vi "GetSegmentBands.vi"(9 "stop frequency":dbl format="%#_6p", 10 "start frequency":dbl format="%#_6p", 11 "sweeps in":T1[](array[typedef]) {"bandwidth" format="%#_6p"; "stop" format="%#_6p"; "start" format="%#_6p"}) -> (3 "sweeps out":T1[](array[typedef]) {"bandwidth" format="%#_6p"; "stop" format="%#_6p"; "start" format="%#_6p"})   [LabVIEW 2017, in "EmsaAnalysis.lvlib"]
uses:
  <vilib>/addons/InsightCM/Devices/Shared/Emsa/EmsaAnalysis/EmsaAnalysis.lvlib
  <vilib>/addons/InsightCM/Devices/Shared/Emsa/EmsaAnalysis/controls/sweepInfo.ctl
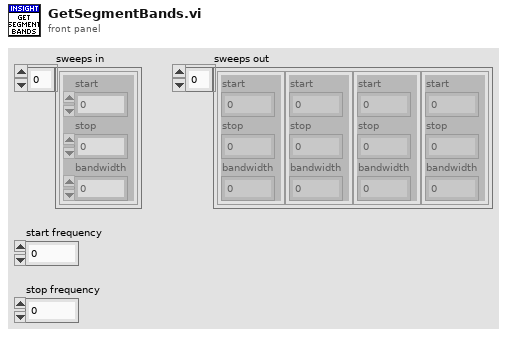
[diagram p1: front panel]
types:
  T1 = typedef "EmsaAnalysis.lvlib/sweepInfo.ctl" = cluster{"start":dbl, "stop":dbl, "bandwidth":dbl}
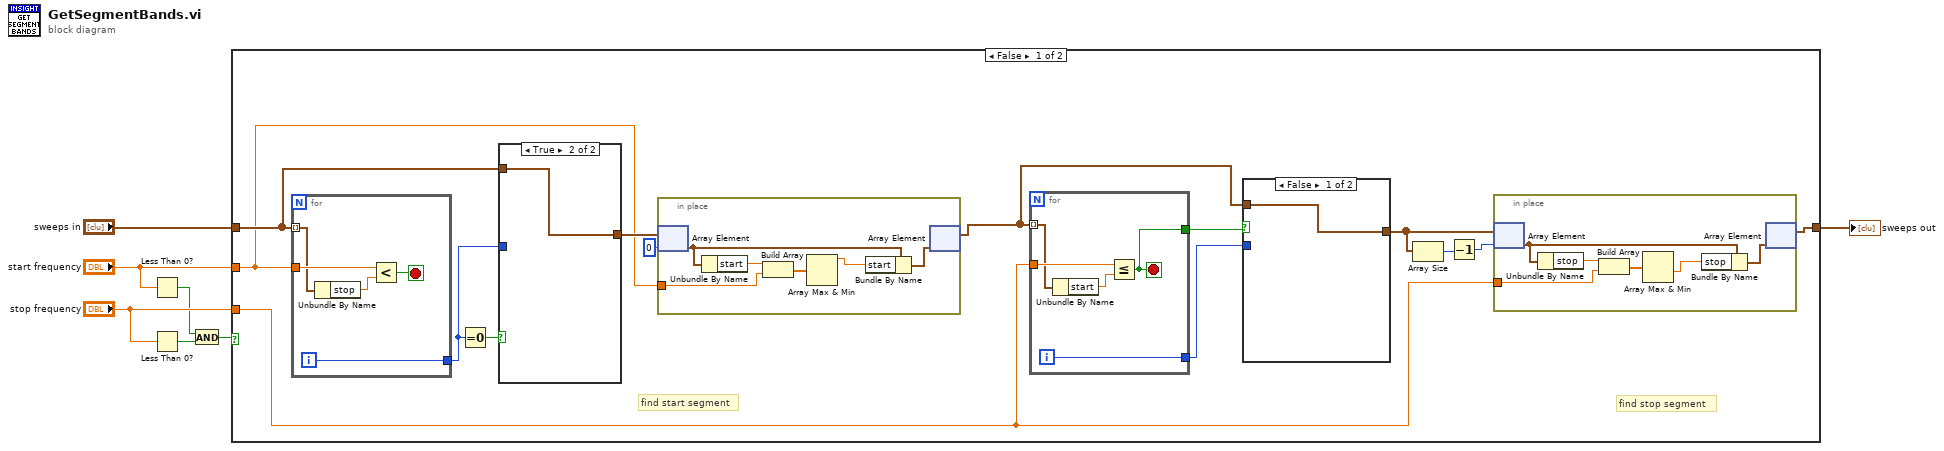
[diagram p0: block diagram]
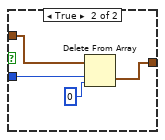
[diagram p2: hidden frame]
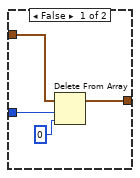
[diagram p3: hidden frame]
diagram:
  n1 = Less Than 0?(x="start frequency") -> (x < 0?=w2:bool)
  n2 = Less Than 0?(x="stop frequency") -> (x < 0?=w1:bool)
  n3 = And(x=w2, y=w1) -> (x .and. y?=w3:bool)
  n4 = case shown="False" w3 {
    tunnel: "sweeps in" -> [w21 w54]
    tunnel: "start frequency" -> [w16 _]
    tunnel: "stop frequency" -> [w14 _]
    tunnel: [w13 w54] -> w7
    frame False {
      # "find stop segment"
      # "find start segment"
      n5 = for {
        tunnel: w21 -> [w51] mode=indexing
        tunnel: w16 -> [w52]
        tunnel: [w49] -> w20
        i -> [w49]
        stop <- w50 stop-if-true
        n6 = Unbundle By Name(w51) -> ("stop"=w53:dbl)
        n7 = Less?(x=w52, y=w53) -> (x < y?=w50:bool)
      }
      n8 = Equal To 0?(x=w20) -> (x = 0?=w19:bool)
      n9 = case shown="True" w19 {
        tunnel: w21 -> [w47 w48]
        tunnel: w20 -> [w45 _]
        tunnel: [w44 w48] -> w18
        frame False {
          n10 = Delete From Array(array=w47, length=w45, index=0) -> (array with subset deleted=w44:T1[])  [unwired: 1 out]
        }
        frame True {
        }
      }
      n11 = in-place {
        in-place-border: w16 -> [w40]
        n12 = in-place-array #1(w18, 0) -> (w43:T1)
        n13 = Unbundle By Name(w43) -> ("start"=w41:dbl)
        n14 = Build Array(w41, w40) -> (w39:dbl[])
        n15 = Array Max & Min(array=w39) -> (max value=w38:dbl)  [unwired: 3 out]
        n16 = Bundle By Name(cluster=w43, "start"=w38) -> (w42:T1)
        n17 = in-place-array #1(w42) -> (w15:T1[])  [unwired: 1 out]
      }
      n18 = for {
        tunnel: w15 -> [w35] mode=indexing
        tunnel: w14 -> [w36]
        tunnel: [w34] -> w9
        tunnel: [w33] -> w8
        i -> [w34]
        stop <- w33 stop-if-true
        n19 = Unbundle By Name(w35) -> ("start"=w37:dbl)
        n20 = Less Or Equal?(x=w36, y=w37) -> (x <= y?=w33:bool)
      }
      n21 = case shown="False" w8 {
        tunnel: w15 -> [w22 w26]
        tunnel: [w22 w25] -> w12
        tunnel: w9 -> [_ w23]
        frame False {
        }
        frame True {
          n22 = Delete From Array(array=w26, length=w23, index=0) -> (deleted portion=w25:T1[])  [unwired: 1 out]
        }
      }
      n23 = Array Size(array=w12) -> (size(s)=w11:i32)
      n24 = Decrement(x=w11) -> (x-1=w10:i32)
      n25 = in-place {
        in-place-border: w14 -> [w29]
        n26 = in-place-array #2(w12, w10) -> (w32:T1)
        n27 = Unbundle By Name(w32) -> ("stop"=w30:dbl)
        n28 = Build Array(w30, w29) -> (w28:dbl[])
        n29 = Array Max & Min(array=w28) -> (min value=w27:dbl)  [unwired: 3 out]
        n30 = Bundle By Name(cluster=w32, "stop"=w27) -> (w31:T1)
        n31 = in-place-array #2(w31) -> (w13:T1[])  [unwired: 1 out]
      }
    }
    frame True {
      # "calculate over the entire band"
    }
  }
  "sweeps out" <- w7
